vi "Method_Const.vi"(4 "Value":u32, 5 "A":T1) -> (1 "Result":T1)   [LabVIEW 2021, in "NOR_U32.lvclass"]
uses:
  NOR_U32.lvclass
  Abs_Type.ctl
  Abs_Types/U32 Integer/Abs_U32 Integer.lvclass
  C:/TSA/LV_Abstract/Source/Functions/Support/Function/Two Terminal/U32/AbsFunc_Two Term_U32.lvclass
  C:/Program Files (x86)/National Instruments/LabVIEW 2021/vi.lib/TSA/Abstract Data Classes/Abs_Types/U32 Integer/Abs_U32 Integer.lvclass
  Support/Function/Two Terminal/U32/AbsFunc_Two Term_U32.lvclass/AbsFunc_Two Term_U32.ctl
  Support/Function/Two Terminal/U32/Properties/Write Numeric A.vi
  Support/Function/Two Terminal/U32/Properties/Write Numeric B.vi
  Constants/Support/U32/Const_U32.lvclass
  C:/Program Files (x86)/National Instruments/LabVIEW 2021/vi.lib/TSA/Abstract Data Classes/Abs_Types/Numeric/Abs_Numeric.lvclass
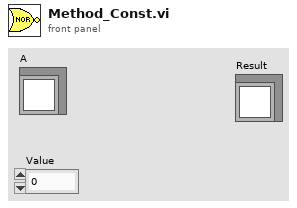
[diagram p1: front panel]
types:
  T1 = typedef "NOR_U32.lvclass/Abs_Type.ctl" = refnum<class "Abs_U32 Integer.lvclass">
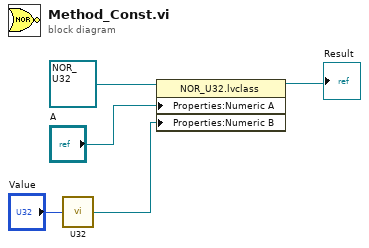
[diagram p0: block diagram]
diagram:
  n1 = call "U32.vi"("Value"="Value") -> ("Constant"=w2:refnum<class "Const_U32.lvclass">)  [unwired: 4 in]
  n2 = property class="NOR_U32.lvclass"(reference=refnum<class "NOR_U32.lvclass"> refnum ("Functions.lvlib:Logic.lvlib:AND.lvclass"), "Properties:Numeric A"="A", "Properties:Numeric B"=w2) -> (reference out=→"Result":refnum<class "NOR_U32.lvclass">)  [unwired: 1 in, 1 out]
